vi "Set_Gain_DUPVA-1-70.vi"(3 "error in":errorcluster, 4 "Status":i32, 5 "Gain [dB]":T1(ring), 6 "index":i32) -> (0 "error out":errorcluster, 1 "Status_out":i32, 2 "index_out":i32)   [LabVIEW 2010, in "FEMTO_LUCI-10.lvlib"]
uses:
  <userlib>/FEMTO/FEMTO_LUCI-10.lvlib
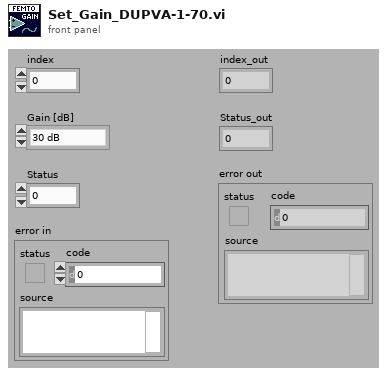
[diagram p1: front panel]
types:
  T1 = enum16{"30 dB", "40 dB", "50 dB", "60 dB", "70 dB"}
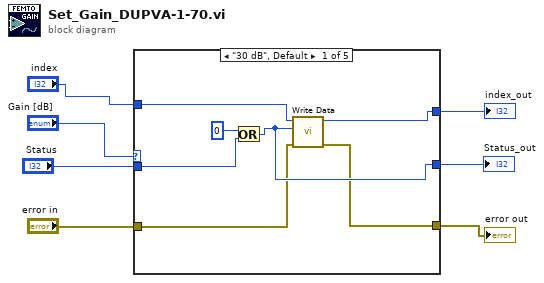
[diagram p0: block diagram]
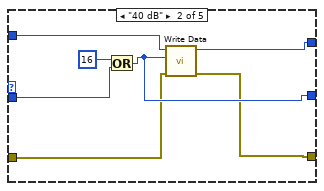
[diagram p2: hidden frame]
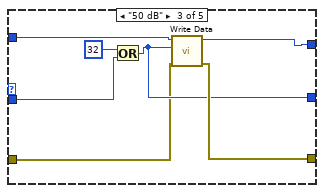
[diagram p3: hidden frame]
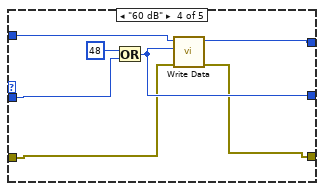
[diagram p4: hidden frame]
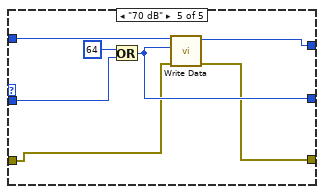
[diagram p5: hidden frame]
diagram:
  n1 = case shown="\"30 dB\", Default" "Gain [dB]" {
    tunnel: [w10 w21 w24 w33 w40] -> w7
    tunnel: "Status" -> [w11 w20 w23 w34 w41]
    tunnel: [w8 w19 w25 w29 w36] -> w5
    tunnel: "error in" -> [w9 w18 w22 w30 w37]
    tunnel: [w12 w17 w26 w32 w39] -> w3
    tunnel: "index" -> [w13 w16 w27 w31 w38]
    frame "30 dB", Default {
      n2 = Or(x=0 ("data_low"), y=w11) -> (x .or. y?=w10:i32)
      n3 = call <userlib>:"Write Data.vi"("error in (no error)"=w9, "data_low"=w10, "index"=w13) -> ("error out"=w8:errorcluster, "index_out"=w12:i32)  [unwired: 1 in, 6 out]
    }
    frame "40 dB" {
      n4 = Or(x=16 ("data_low"), y=w20) -> (x .or. y?=w21:i32)
      n5 = call <userlib>:"Write Data.vi"("error in (no error)"=w18, "data_low"=w21, "index"=w16) -> ("error out"=w19:errorcluster, "index_out"=w17:i32)  [unwired: 1 in, 6 out]
    }
    frame "50 dB" {
      n6 = Or(x=32 ("data_low"), y=w23) -> (x .or. y?=w24:i32)
      n7 = call <userlib>:"Write Data.vi"("error in (no error)"=w22, "data_low"=w24, "index"=w27) -> ("error out"=w25:errorcluster, "index_out"=w26:i32)  [unwired: 1 in, 6 out]
    }
    frame "60 dB" {
      n8 = Or(x=48 ("data_low"), y=w34) -> (x .or. y?=w33:i32)
      n9 = call <userlib>:"Write Data.vi"("error in (no error)"=w30, "data_low"=w33, "index"=w31) -> ("error out"=w29:errorcluster, "index_out"=w32:i32)  [unwired: 1 in, 6 out]
    }
    frame "70 dB" {
      n10 = Or(x=64 ("data_low"), y=w41) -> (x .or. y?=w40:i32)
      n11 = call <userlib>:"Write Data.vi"("error in (no error)"=w37, "data_low"=w40, "index"=w38) -> ("error out"=w36:errorcluster, "index_out"=w39:i32)  [unwired: 1 in, 6 out]
    }
  }
  "index_out" <- w3
  "error out" <- w5
  "Status_out" <- w7
